vi "Config Load Auton Globals.vi"(11 "refnum":T1) -> (3 "refnum 2":T1)   [LabVIEW 2012]
uses:
  <vilib>/Utility/config.llb/Config Data RefNum.ctl
  <vilib>/Utility/config.llb/Read Key (Double).vi
  Auton Globals.vi
  <vilib>/Utility/config.llb/NI_LVConfig.lvlib
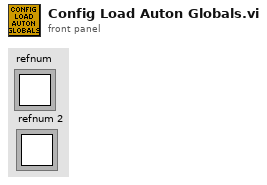
[diagram p1: front panel]
types:
  T1 = typedef "NI_LVConfig.lvlib/Config Data RefNum.ctl" = refnum<k1>
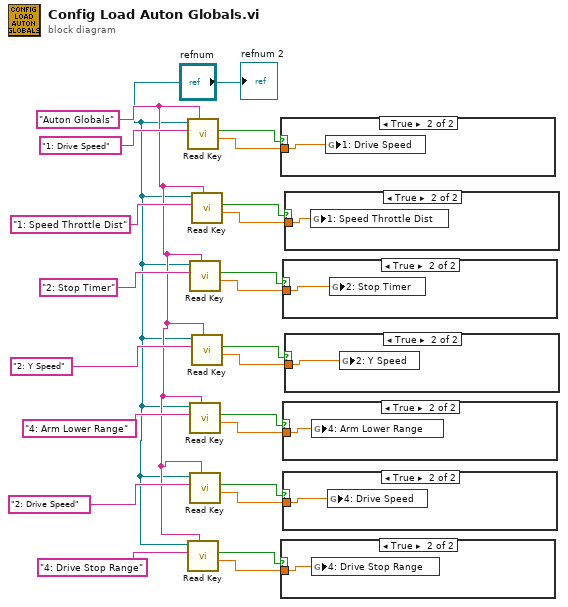
[diagram p0: block diagram]
diagram:
  w2 = "Auton Globals"
  n1 = call-poly <vilib>:"Read Key.vi"("section"=w2, "key"="1: Drive Speed", "refnum"="refnum") -> ("value"=w23:dbl, "found?"=w21:bool)  [unwired: 5 in, 2 out]
  n2 = call-poly <vilib>:"Read Key.vi"("section"=w2, "key"="4: Drive Stop Range", "refnum"="refnum") -> ("value"=w5:dbl, "found?"=w3:bool)  [unwired: 5 in, 2 out]
  n3 = call-poly <vilib>:"Read Key.vi"("section"=w2, "key"="2: Stop Timer", "refnum"="refnum") -> ("value"=w17:dbl, "found?"=w15:bool)  [unwired: 5 in, 2 out]
  n4 = call-poly <vilib>:"Read Key.vi"("section"=w2, "key"="4: Arm Lower Range", "refnum"="refnum") -> ("value"=w12:dbl, "found?"=w14:bool)  [unwired: 5 in, 2 out]
  n5 = call-poly <vilib>:"Read Key.vi"("section"=w2, "key"="2: Drive Speed", "refnum"="refnum") -> ("value"=w6:dbl, "found?"=w8:bool)  [unwired: 5 in, 2 out]
  n6 = call-poly <vilib>:"Read Key.vi"("section"=w2, "key"="1: Speed Throttle Dist", "refnum"="refnum") -> ("value"=w18:dbl, "found?"=w20:bool)  [unwired: 5 in, 2 out]
  n7 = call-poly <vilib>:"Read Key.vi"("section"=w2, "key"="2: Y Speed", "refnum"="refnum") -> ("value"=w11:dbl, "found?"=w9:bool)  [unwired: 5 in, 2 out]
  n8 = case shown="True" w21 {
    tunnel: w23 -> [_ w24]
    frame False {
    }
    frame True {
      n9 = global write "Auton Globals.vi" "1: Drive Speed"(w24) -> ()
    }
  }
  n10 = case shown="True" w3 {
    tunnel: w5 -> [_ w25]
    frame False {
    }
    frame True {
      n11 = global write "Auton Globals.vi" "4: Drive Stop Range"(w25) -> ()
    }
  }
  n12 = case shown="True" w15 {
    tunnel: w17 -> [_ w26]
    frame False {
    }
    frame True {
      n13 = global write "Auton Globals.vi" "2: Stop Timer"(w26) -> ()
    }
  }
  n14 = case shown="True" w14 {
    tunnel: w12 -> [_ w27]
    frame False {
    }
    frame True {
      n15 = global write "Auton Globals.vi" "4: Arm Lower Range"(w27) -> ()
    }
  }
  n16 = case shown="True" w8 {
    tunnel: w6 -> [_ w28]
    frame False {
    }
    frame True {
      n17 = global write "Auton Globals.vi" "4: Drive Speed"(w28) -> ()
    }
  }
  n18 = case shown="True" w20 {
    tunnel: w18 -> [_ w29]
    frame False {
    }
    frame True {
      n19 = global write "Auton Globals.vi" "1: Speed Throttle Dist"(w29) -> ()
    }
  }
  n20 = case shown="True" w9 {
    tunnel: w11 -> [_ w30]
    frame False {
    }
    frame True {
      n21 = global write "Auton Globals.vi" "2: Y Speed"(w30) -> ()
    }
  }
  "refnum 2" <- "refnum"
